vi "Builder.Cast Command.Build.vi"(1 "command":T2) -> (0 "build/parse command":T1)   [LabVIEW 2016, in "DSF.Engine.lvlib" / "Builder.lvclass"]
uses:
  Builder.lvclass
  Interface/DSF.Engine.Interface.Builder.Command Data.ctl
  Interface/DSF.Engine.Interface.Builder.Command.ctl
  Builder.Command.Build-Parse.ctl
  Interface/DSF.Engine.Interface.Builder.lvclass
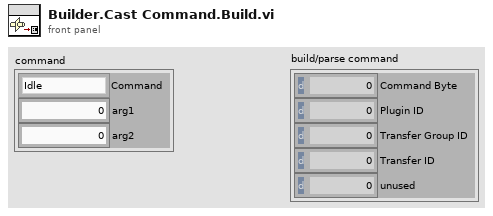
[diagram p1: front panel]
types:
  T1 = typedef "DSF.Engine.lvlib/Builder.lvclass/Builder.Command.Build-Parse.ctl" = cluster{"Command Byte":u8, "Plugin ID":i32, "Transfer Group ID":i32, "Transfer ID":i32, "unused":i32}
  T2 = typedef "DSF.Engine.lvlib/DSF.Engine.Interface.Builder.lvclass/DSF.Engine.Interface.Builder.Command Data.ctl" = cluster{"Command":T3, "arg1":u64, "arg2":u64}
  T3 = typedef "DSF.Engine.lvlib/DSF.Engine.Interface.Builder.lvclass/DSF.Engine.Interface.Builder.Command.ctl" = enum8{"Idle", "Initialize", "Build Buffer", "Parse Buffer", "Shutdown"}
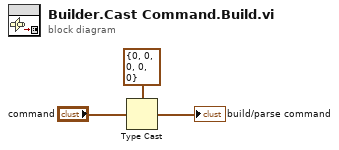
[diagram p0: block diagram]
diagram:
  n1 = Type Cast(type=T1 {"Command Byte"=0, "Plugin ID"=0, "Transfer Group ID"=0, "Transfer ID"=0, "unused"=0} ("build command"), x="command") -> (*(type *) &x=→"build/parse command":T1)
